vi "Create Arduino Detectors.vi"(8 "error in (no error)":errorcluster, 11 "Controller in":refnum<class "Controller.lvclass">) -> (0 "error out":errorcluster, 3 "Controller out":refnum<class "Controller.lvclass">)   [LabVIEW 2019, in "Controller.lvlib" / "Controller.lvclass"]
uses:
  Controller.lvclass
  C:/Program Files (x86)/National Instruments/LabVIEW 2019/vi.lib/ActorFramework/Actor/Actor.lvclass
  Detector Actor/Detector Actor/Detector Actor.lvclass
  Sensors/Arduino/Arduino Detector.lvclass
  C:/LabVIEW Sources/Muon Detector/Sensors/Detector/Muon Detector.lvclass
  Sensors/Arduino/Arduino Detector.lvclass/Arduino Detector.ctl
  Detector Actor/Detector Actor/Detector Actor.lvclass/Detector Actor.ctl
  2e910c9f-3303-4c6c-8fa8-2d3f1a59dc2a.vi
  <vilib>/ActorFramework/Actor/Actor.lvclass
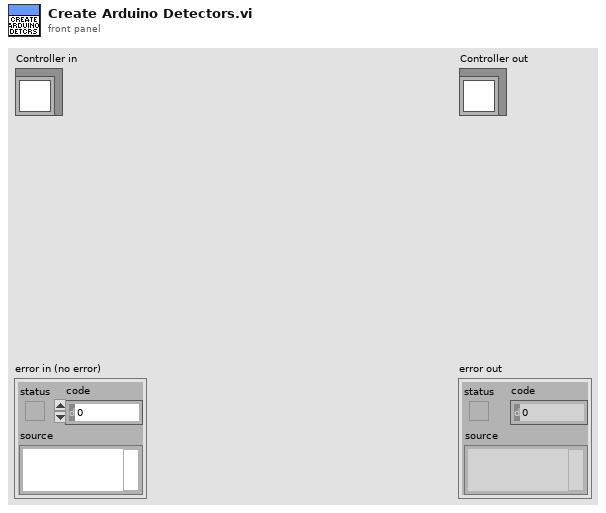
[diagram p1: front panel]
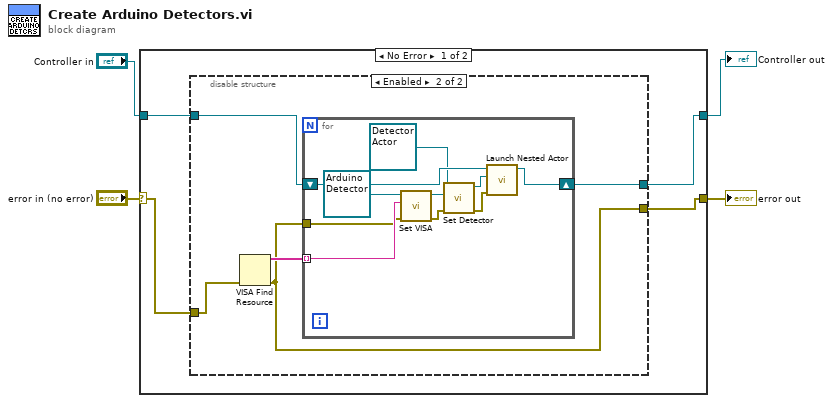
[diagram p0: block diagram]
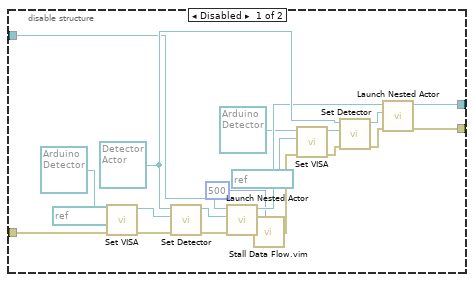
[diagram p2: hidden frame]
diagram:
  n1 = case shown="No Error" "error in (no error)" {
    selector: "error in (no error)" -> [w5 w46]
    tunnel: [w6 w46] -> w3
    tunnel: [w8 w45] -> w1
    tunnel: "Controller in" -> [w7 w45]
    frame No Error {
      n2 = disable-structure shown="Enabled" {
        disable-tunnel: [w25 w31] -> w8
        disable-tunnel: w7 -> [w24 w30]
        disable-tunnel: [w23 w32] -> w6
        disable-tunnel: w5 -> [w20 w34]
        frame Disabled {
          w29 = refnum<class "Detector Actor.lvclass"> refnum ("Detector Actor.lvlib:Detector Actor.lvclass")
          n3 = call "Set VISA.vi"("error in (no error)"=w20, "VISA"=refnum<visa-resource-name> "COM6", "Arduino Detector in"=refnum<class "Arduino Detector.lvclass"> refnum ("Arduino Detector.lvclass")) -> ("error out"=w19:errorcluster, "Arduino Detector out"=w18:refnum<class "Arduino Detector.lvclass">)  [unwired: 7 in]
          n4 = call "Set Detector.vi"("error in (no error)"=w19, "Muon Detector"=w18, "Detector Actor in"=w29) -> ("error out"=w22:errorcluster, "Detector Actor out"=w28:refnum<class "Detector Actor.lvclass">)  [unwired: 7 in]
          n5 = call <vilib>:"Launch Nested Actor.vi"("error in (no error)"=w22, "Nested Actor"=w28, "Caller Actor in"=w24) -> ("error out"=w11:errorcluster, "Caller Actor out"=w26:refnum<class "Controller.lvclass">)  [unwired: 6 in, 1 out]
          n6 = call "Stall Data Flow.vim"("value in"=w11, "milliseconds to wait"=u32 500) -> ("value out"=w10:errorcluster)  [unwired: 1 out]
          n7 = call "Set VISA.vi"("error in (no error)"=w10, "VISA"=refnum<visa-resource-name> "COM5", "Arduino Detector in"=refnum<class "Arduino Detector.lvclass"> refnum ("Arduino Detector.lvclass")) -> ("error out"=w13:errorcluster, "Arduino Detector out"=w12:refnum<class "Arduino Detector.lvclass">)  [unwired: 7 in]
          n8 = call "Set Detector.vi"("error in (no error)"=w13, "Muon Detector"=w12, "Detector Actor in"=w29) -> ("error out"=w21:errorcluster, "Detector Actor out"=w27:refnum<class "Detector Actor.lvclass">)  [unwired: 7 in]
          n9 = call <vilib>:"Launch Nested Actor.vi"("error in (no error)"=w21, "Nested Actor"=w27, "Caller Actor in"=w26) -> ("error out"=w23:errorcluster, "Caller Actor out"=w25:refnum<class "Controller.lvclass">)  [unwired: 6 in, 1 out]
        }
        frame Enabled {
          n10 = VISA Find Resource(8:w34) -> (0:w32:errorcluster, 3:w33:string[])  [unwired: 2 in, 1 out]
          n11 = for {
            tunnel: w33 -> [w40] mode=indexing
            tunnel: w32 -> [w39]
            shift-right: [w38] -> w31
            shift-left: w30 -> [w37]
            n12 = call "Set VISA.vi"("error in (no error)"=w39, "VISA"=w40, "Arduino Detector in"=refnum<class "Arduino Detector.lvclass"> refnum ("Arduino Detector.lvclass")) -> ("error out"=w42:errorcluster, "Arduino Detector out"=w36:refnum<class "Arduino Detector.lvclass">)  [unwired: 7 in]
            n13 = call "Set Detector.vi"("error in (no error)"=w42, "Muon Detector"=w36, "Detector Actor in"=refnum<class "Detector Actor.lvclass"> refnum ("Detector Actor.lvlib:Detector Actor.lvclass")) -> ("error out"=w43:errorcluster, "Detector Actor out"=w44:refnum<class "Detector Actor.lvclass">)  [unwired: 7 in]
            n14 = call <vilib>:"Launch Nested Actor.vi"("error in (no error)"=w43, "Nested Actor"=w44, "Caller Actor in"=w37) -> ("Caller Actor out"=w38:refnum<class "Controller.lvclass">)  [unwired: 6 in, 2 out]
          }
        }
      }
    }
    frame Error {
    }
  }
  "error out" <- w3
  "Controller out" <- w1
